vi "Is Valid Linkage.vi"(8 "error in (no error)":errorcluster, 10 "Channel Refnum":T1 format="%.0x", 11 "Variable Name":string) -> (0 "error out":errorcluster, 2 "Is Valid Linkage?":bool, 3 "Linkage":cluster{"Variable Name":string, "GUID":string})   [LabVIEW 2020, in "Instrument Addon Scripting API.lvlib"]
uses:
  Instrument Addon Scripting API.lvlib
  <vilib>/NI VeriStand/Custom Device API/Custom Device Item Ref.ctl
  Addon/Addon Shared/SubVIs/Constants.vi
  <vilib>/NI VeriStand/Custom Device API/Get Item Property (String).vi
  <vilib>/NI VeriStand/Custom Device API/Custom Device API.lvlib
  Addon/Addon Shared/Instrument Addon Shared.lvlib
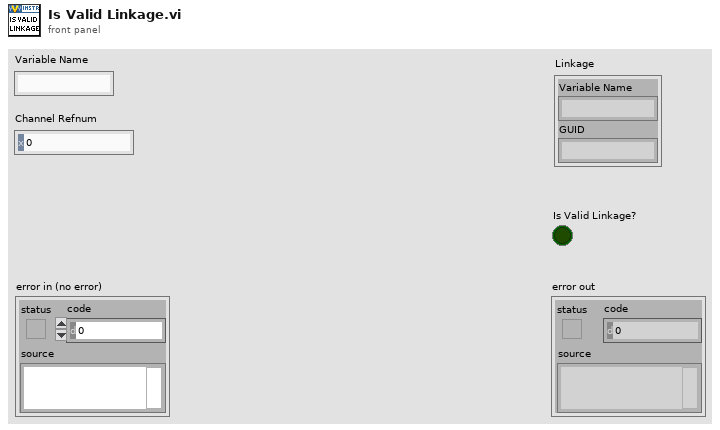
[diagram p1: front panel]
types:
  T1 = typedef "Custom Device API.lvlib/Custom Device Item Ref.ctl" = u64
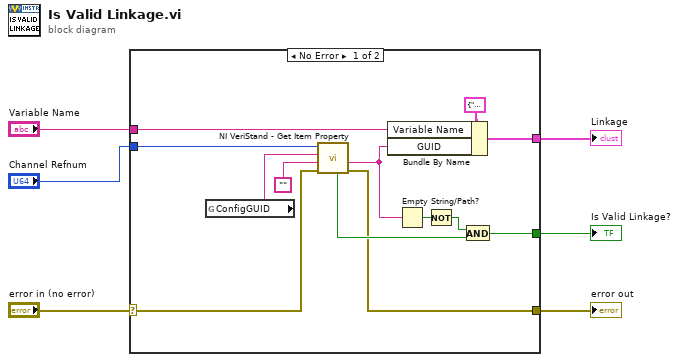
[diagram p0: block diagram]
diagram:
  n1 = case shown="No Error" "error in (no error)" {
    selector: "error in (no error)" -> [w7 w20]
    tunnel: [w12 w20] -> w6
    tunnel: [w11 _] -> w5
    tunnel: [w10 _] -> w4
    tunnel: "Variable Name" -> [w9 _]
    tunnel: "Channel Refnum" -> [w8 _]
    frame No Error {
      n2 = global read "Constants.vi" "ConfigGUID"() -> (w19:string)
      n3 = call-poly <vilib>:"NI VeriStand - Get Item Property.vi"("error in (no error)"=w7, "Default Value"="", "Property Name"=w19, "Item Ref in"=w8) -> ("error out"=w12:errorcluster, "Value"=w13:string, "Found?"=w17:bool)  [unwired: 4 in, 1 out]
      n4 = Bundle By Name(cluster=cluster{"Variable Name":string, "GUID":string} {"Variable Name"="", "GUID"=""}, "Variable Name"=w9, "GUID"=w13) -> (w10:cluster{"Variable Name":string, "GUID":string})
      n5 = Empty String/Path?(string/path=w13) -> (empty?=w16:bool)
      n6 = Not(x=w16) -> (.not. x?=w15:bool)
      n7 = And(x=w15, y=w17) -> (x .and. y?=w11:bool)
    }
    frame Error {
    }
  }
  "error out" <- w6
  "Is Valid Linkage?" <- w5
  "Linkage" <- w4
